vi "Uninitialize.vi"(8 "error in":errorcluster) -> (0 "error out":errorcluster)   [LabVIEW 2017, in "JKI Simple Localization.lvlib"]
doc: "Removes all VIs from registry, deletes the current language and the dictionary."
uses:
  JKI Simple Localization.lvlib
  Definitions/Private/Localization FGV Action -- Enum.ctl
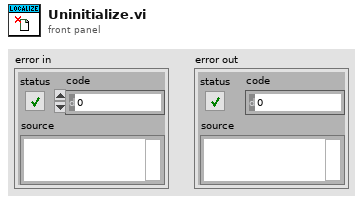
[diagram p1: front panel]
types:
  T1 = typedef "JKI Simple Localization.lvlib/Localization FGV Action -- Enum.ctl" = enum16{"Read Dictionary", "Translate VIs", "Register VI", "Get Languages", "Translate Phrase", "Translate VI", "Unregister"}
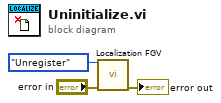
[diagram p0: block diagram]
diagram:
  n1 = call "Localization FGV.vi"("Action"=Localization_FGV_Action_--_Enum."Unregister", "error in"="error in") -> ("error out"=→"error out":errorcluster)  [unwired: 9 in, 4 out]
